vi "Modem Status Read Data.vi"(8 "error in (no error)":errorcluster, 11 "VISA Refnum in":refnum<visa-resource-name>) -> (0 "error out":errorcluster, 1 "Failed":bool, 2 "Msg Body":string, 3 "VISA Refnum out":refnum<visa-resource-name>)   [LabVIEW 2011]
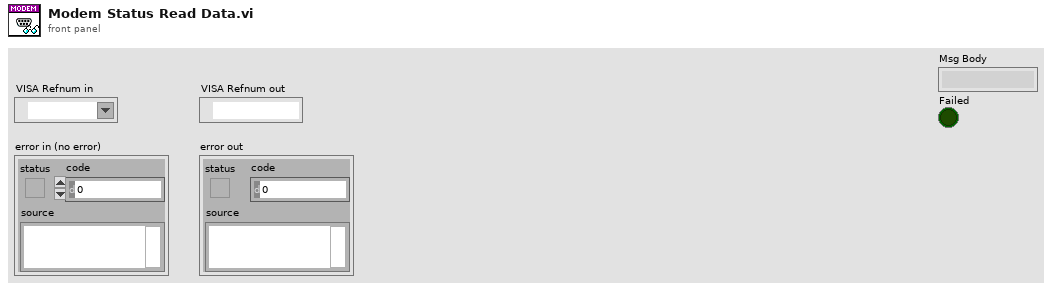
[diagram p1: front panel]
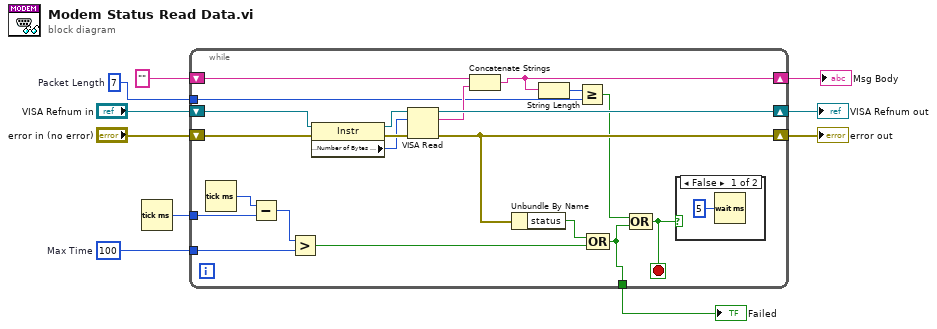
[diagram p0: block diagram]
diagram:
  w2 = 7  # Packet Length
  w4 = u32 100  # Max Time
  n1 = Tick Count (ms)() -> (millisecond timer value=w5:u32)
  n2 = while {
    shift-right: [w28] -> w3
    shift-left: "" -> [w30]
    tunnel: w5 -> [w20]
    tunnel: w4 -> [w18]
    tunnel: w2 -> [w14]
    shift-right: [w17] -> w9
    shift-left: "error in (no error)" -> [w24]
    shift-right: [w31] -> w10
    shift-left: "VISA Refnum in" -> [w26]
    tunnel: [w11] -> w1
    stop <- w12 stop-if-true
    n3 = Tick Count (ms)() -> (millisecond timer value=w21:u32)
    n4 = Subtract(x=w21, y=w20) -> (x-y=w19:u32)
    n5 = Greater?(x=w19, y=w18) -> (0:w15:bool)
    n6 = property class="Instr"(reference=w26, error in=w24) -> (reference out=w25:refnum<visa-resource-name>, error out=w23:errorcluster, "Serial Settings:Number of Bytes at Serial Port"=w22:u32)
    n7 = VISA Read(VISA resource name=w25, byte count=w22, error in (no error)=w23) -> (VISA resource name out=w31:refnum<visa-resource-name>, read buffer=w29:string, error out=w17:errorcluster)  [unwired: 1 out]
    n8 = Concatenate Strings(w30, w29) -> (w28:string)
    n9 = Unbundle By Name(w17) -> ("status"=w16:bool)
    n10 = String Length(string=w28) -> (length=w27:i32)
    n11 = Greater Or Equal?(x=w27, y=w14) -> (x >= y?=w13:bool)
    n12 = Compound Arithmetic op=OR(w16, w15) -> (w11:bool)
    n13 = Compound Arithmetic op=OR(w13, w11) -> (w12:bool)
    n14 = case shown="False" w12 {
      frame False {
        n15 = Wait (ms)(milliseconds to wait=u32 5) -> ()  [unwired: 1 out]
      }
      frame True {
      }
    }
  }
  "VISA Refnum out" <- w10
  "error out" <- w9
  "Msg Body" <- w3
  "Failed" <- w1
